vi "Get Data Log Directory Settings.vi"(8 "error in":errorcluster, 11 "File Ref in":T1 format="%.0x") -> (0 "error out":errorcluster, 1 "Timestamp":bool, 2 "File Path":path, 3 "File Ref Out":T1 format="%.0x", 4 "Archive Files":bool, 5 "Name":string, 6 "Archive Log Directory":path, 7 "Log Directory":path)   [LabVIEW 2018, in "Embedded Data Logger Engine.lvlib"]
uses:
  <vilib>/NI Veristand/Custom Device API/Custom Device Item Ref.ctl
  Shared/Constants.vi
  <vilib>/NI Veristand/Custom Device API/Get Item Property (String Array).vi
  <vilib>/NI Veristand/Custom Device API/Get Item Property (Boolean).vi
  Embedded Data Logger Engine.lvlib
  <vilib>/NI Veristand/Custom Device API/Custom Device API.lvlib
  Shared/Embedded Data Logger Shared.lvlib
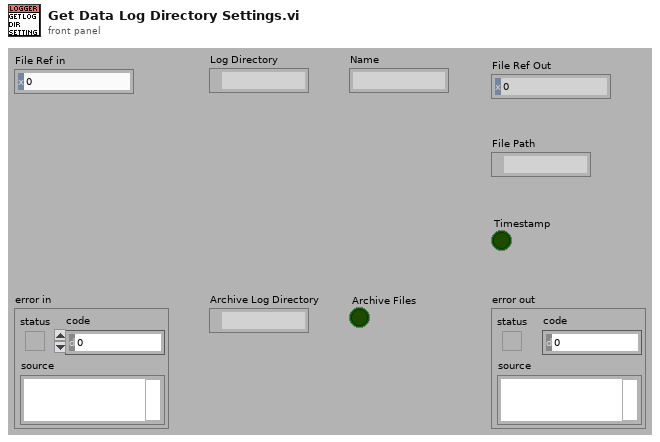
[diagram p1: front panel]
types:
  T1 = typedef "Custom Device API.lvlib/Custom Device Item Ref.ctl" = u64
  T2 = typedef "Custom Device API.lvlib/Custom Device Item Info.ctl" = cluster{"Name":string, "Is Channel":bool, "GUID":string, "Is Waveform":bool}
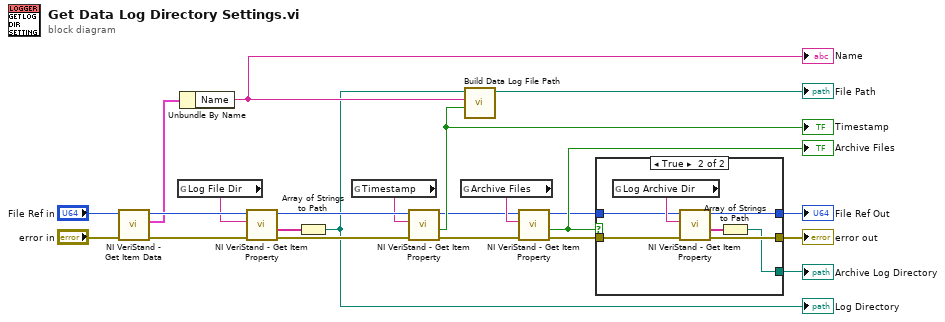
[diagram p0: block diagram]
diagram:
  n1 = call <vilib>:"NI VeriStand - Get Item Data.vi"("error in (no error)"="error in", "Item Ref in"="File Ref in") -> ("error out"=w20:errorcluster, "Item Info"=w16:T2, "Item Ref out"=w22:T1)  [unwired: 7 out]
  n2 = global read "Constants.vi" "Log File Dir"() -> (w11:string)
  n3 = Unbundle By Name(w16) -> ("Name"=w18:string)
  "Name" <- w18
  n4 = call-poly <vilib>:"NI VeriStand - Get Item Property.vi"("error in (no error)"=w20, "Property Name"=w11, "Item Ref in"=w22) -> ("error out"=w21:errorcluster, "Value"=w13:string[], "Item Ref out"=w23:T1)  [unwired: 1 in, 5 out]
  n5 = Array of Strings to Path(0:w13) -> (2:w12:path)  [unwired: 1 in]
  "Log Directory" <- w12
  n6 = global read "Constants.vi" "Timestamp"() -> (w10:string)
  n7 = call-poly <vilib>:"NI VeriStand - Get Item Property.vi"("error in (no error)"=w21, "Property Name"=w10, "Item Ref in"=w23) -> ("error out"=w3:errorcluster, "Value"=w17:bool, "Item Ref out"=w4:T1)  [unwired: 1 in, 5 out]
  "Timestamp" <- w17
  n8 = global read "Constants.vi" "Archive Files"() -> (w9:string)
  n9 = call "Build Data Log File Path.vi"("Timestamp"=w17, "Name"=w18, "Log File Directory"=w12) -> ("appended path"=→"File Path":path)  [unwired: 7 in, 1 out]
  n10 = call-poly <vilib>:"NI VeriStand - Get Item Property.vi"("error in (no error)"=w3, "Property Name"=w9, "Item Ref in"=w4) -> ("error out"=w1:errorcluster, "Value"=w5:bool, "Item Ref out"=w2:T1)  [unwired: 1 in, 5 out]
  "Archive Files" <- w5
  n11 = case shown="True" w5 {
    tunnel: w2 -> [w25 w30]
    tunnel: [w25 w29] -> w8
    tunnel: w1 -> [w24 w28]
    tunnel: [w24 w27] -> w7
    tunnel: [_ w26] -> w6
    frame False {
    }
    frame True {
      n12 = global read "Constants.vi" "Log Archive Dir"() -> (w32:string)
      n13 = call-poly <vilib>:"NI VeriStand - Get Item Property.vi"("error in (no error)"=w28, "Property Name"=w32, "Item Ref in"=w30) -> ("error out"=w27:errorcluster, "Value"=w31:string[], "Item Ref out"=w29:T1)  [unwired: 1 in, 5 out]
      n14 = Array of Strings to Path(0:w31) -> (2:w26:path)  [unwired: 1 in]
    }
  }
  "File Ref Out" <- w8
  "error out" <- w7
  "Archive Log Directory" <- w6
